vi "MODES.vi"(9 "Definitions":T1(array[cluster])=[{"Name"="LPF2-DETECT", "Format"={"# Datasets"=1, "Data Type"=0, "Figures"=3, "Decimals"=0}, "Raw"={"Min"=0.0, "Max"=10.0}, "Pct"={"Min"=0.0, "Max"=100.0}, "SI"={"Min"=0.0, "Max"=10.0}, "Symbol"="", "Funct Map"={"In"=16, "Out"=0}, "view?"=TRUE}, {"Name"="LPF2-COUNT", "Format"={"# Datasets"=1, "Data Type"=2, "Figures"=4, "Decimals"=0}, "Raw"={"Min"=0.0, "Max"=100.0}, "Pct"={"Min"=0.0, "Max"=100.0}, "SI"={"Min"=0.0, "Max"=100.0}, "Symbol"="CNT", "Funct Map"={"In"=16, "Out"=0}, "view?"=TRUE}, {"Name"="LPF2-CAL", "Format"={"# Datasets"=3, "Data Type"=1, "Figures"=3, "Decimals"=0}, "Raw"={"Min"=0.0, "Max"=1023.0}, "Pct"={"Min"=0.0, "Max"=100.0}, "SI"={"Min"=0.0, "Max"=1023.0}, "Symbol"="RAW", "Funct Map"={"In"=16, "Out"=0}, "view?"=FALSE}] {"Format"."Data Type" items=["DATA8", "DATA16", "DATA32", "DATAF"]; "Funct Map"."In" items=["ABSOLUTE"=16, "RELATIVE"=8, "DISCRETE"=4]}, 11 "Python in":string="import machine, utime\n\ntx = machine.Pin('Y9', machine.Pin.OUT)\nrx = machine.Pin('Y10', machine.Pin.IN)\ntx.value(b'\\x00')\nutime.sleep_ms(500)\ntx.value(1)\n\nuart = machine.UART(3)\nuart.init(baudrate=2400, bits=8, parity=None, stop=1)\n\nuart.write(0)\nuart.write(b'\\x40\\x23\\x9C')\n") -> (3 "Python out":string="import machine, utime\n\ntx = machine.Pin('Y9', machine.Pin.OUT)\nrx = machine.Pin('Y10', machine.Pin.IN)\ntx.value(b'\\x00')\nutime.sleep_ms(500)\ntx.value(1)\n\nuart = machine.UART(3)\nuart.init(baudrate=2400, bits=8, parity=None, stop=1)\n\nuart.write(0)\nuart.write(b'\\x40\\x23\\x9C')\nuart.write(b'\\x49\\x00\\x00\\xB6')\n")   [LabVIEW 2016]
panel:
  out "Modes":u8[](array[numeric])
  out "bytes added":u8[](array[numeric])=[73, 0, 0, 182] format="%.0x"
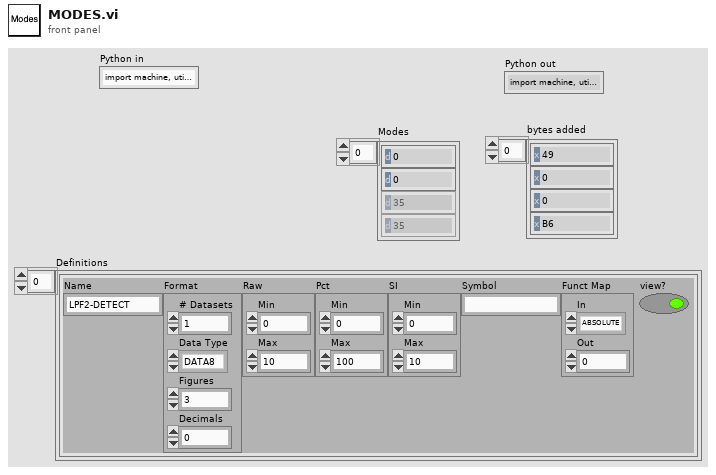
[diagram p1: front panel]
types:
  T1 = cluster{"Name":string, "Format":cluster{"# Datasets":u8, "Data Type":u8, "Figures":u8, "Decimals":u8}, "Raw":cluster{"Min":dbl, "Max":dbl}, "Pct":cluster{"Min":dbl, "Max":dbl}, "SI":cluster{"Min":dbl, "Max":dbl}, "Symbol":string, "Funct Map":cluster{"In":u8, "Out":u8}, "view?":bool}[]
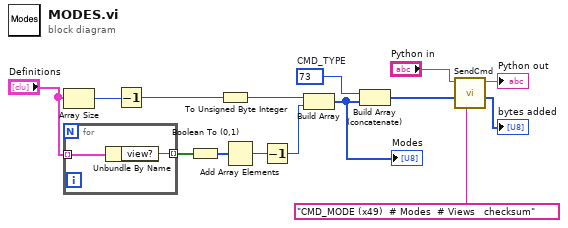
[diagram p0: block diagram]
diagram:
  w15 = u8 73  # CMD_TYPE
  n1 = Array Size(array="Definitions") -> (size(s)=w10:i32)
  n2 = for {
    tunnel: "Definitions" -> [w17] mode=indexing
    tunnel: [w16] -> w8 mode=indexing
    n3 = Unbundle By Name(w17) -> ("view?"=w16:bool)
  }
  n4 = Decrement(x=w10) -> (x-1=w9:i32)
  n5 = Boolean To (0,1)(Boolean=w8) -> (0, 1=w7:i16[])
  n6 = To Unsigned Byte Integer(number=w9) -> (unsigned 8bit integer=w2:u8)
  n7 = Add Array Elements(numeric array=w7) -> (sum=w6:i16)
  n8 = Decrement(x=w6) -> (x-1=w5:i16)
  n9 = Build Array(w2, w5) -> (w3:i16[])
  "Modes" <- w3
  n10 = Build Array (concatenate)(w15, w3) -> (w12:i16[])
  n11 = call "SendCmd.vi"("Comment"="CMD_MODE (x49)  # Modes  # Views   checksum", "Array In"=w12, "Python in"="Python in") -> ("Array Sent"=→"bytes added":u8[], "Python out"=→"Python out":string)  [unwired: 7 in]
